vi "AB_User_Log_Output_Item.vi"(8 "error in (no error)":errorcluster, 11 "outputFilePaths":path[](array[path])) -> (0 "error out":errorcluster)   [LabVIEW 2020]
uses:
  <vilib>/AppBuilder/logging/AB_Log_File_Action.ctl
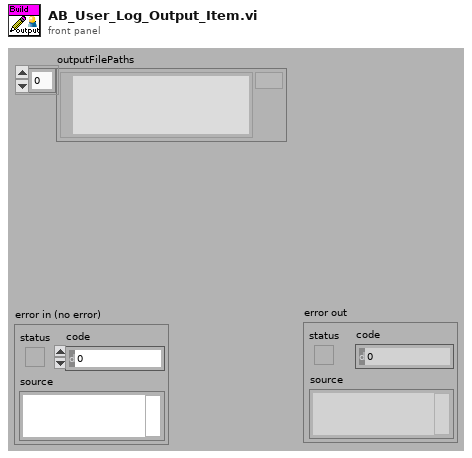
[diagram p1: front panel]
types:
  T1 = typedef "AB_Log_File_Action.ctl" = enum16{"write", "open", "close"}
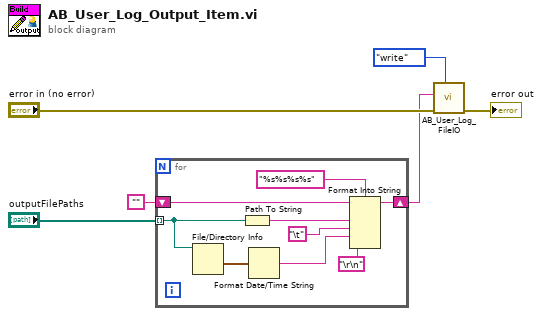
[diagram p0: block diagram]
diagram:
  n1 = for {
    tunnel: "outputFilePaths" -> [w9] mode=indexing
    shift-right: [w12] -> w3
    shift-left: "" -> [w8]
    n2 = File/Directory Info(path=w9) -> (last mod=w15:timestamp)  [unwired: 1 in, 6 out]
    n3 = Path To String(path=w9) -> (string=w13:string)
    n4 = Format Date/Time String(seconds (now)=w15) -> (date/time string=w11:string)  [unwired: 2 out]
    n5 = Format Into String(format string="%s%s%s%s", initial string=w8, w13, "\t", w11, "\r\n") -> (resulting string=w12:string)  [unwired: 1 in, 1 out]
  }
  n6 = call <vilib>:"AB_User_Log_FileIO.vi"("fileAction"=AB_Log_File_Action."write", "error in (no error)"="error in (no error)", "data"=w3) -> ("error out"=→"error out":errorcluster)  [unwired: 2 in, 6 out]
